vi "IntakeStateController.vi"(1 "Selected State (In)":string) -> (0 "Selected State (Out)":string)   [LabVIEW 2019]
doc: "This VI makes all decisions related to the ball intake including both intake deployment and intake speed."
uses:
  dsinstructions.vi
  outputs.vi
panel:
  in  "Intake_Speed":dbl=1.0
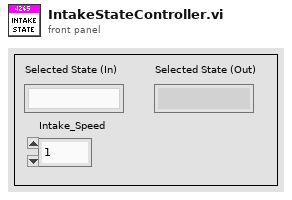
[diagram p1: front panel]
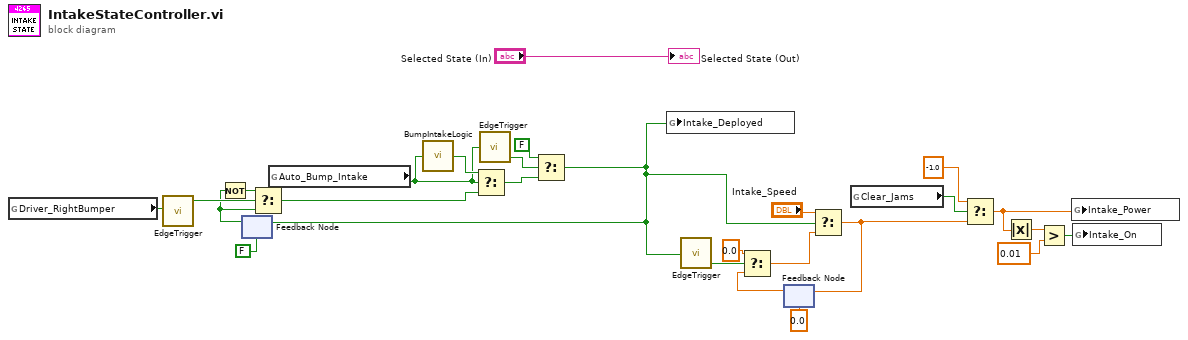
[diagram p0: block diagram]
diagram:
  n1 = global read "dsinstructions.vi" "Driver_RightBumper"() -> (w10:bool)
  n2 = call "EdgeTrigger.vi"("Input Signal"=w10) -> ("Rising Edge Trigger"=w26:bool)  [unwired: 2 out]
  n3 = feedback #1(FALSE ("Intake_On")) -> (w24:bool)
  n4 = Not(x=w24) -> (.not. x?=w23:bool)
  n5 = Select(t=w23, s=w26, f=w24) -> (s? t:f=w9:bool)
  n6 = global read "dsinstructions.vi" "Auto_Bump_Intake"() -> (w6:bool)
  n7 = call "BumpIntakeLogic.vi"("Initiate"=w6) -> ("Auto_Bump_Intake"=w8:bool)
  n8 = Select(t=w8, s=w6, f=w9) -> (s? t:f=w5:bool)
  n9 = call "EdgeTrigger.vi"("Input Signal"=w6) -> ("Falling Edge Trigger"=w7:bool)  [unwired: 2 out]
  n10 = Select(t=FALSE, s=w7, f=w5) -> (s? t:f=w2:bool)
  n11 = feedback-in #1(w2) -> ()
  n12 = global write "outputs.vi" "Intake_Deployed"(w2) -> ()
  n13 = call "EdgeTrigger.vi"("Input Signal"=w2) -> ("Falling Edge Trigger"=w20:bool)  [unwired: 2 out]
  n14 = feedback #2(0.0 ("f")) -> (w18:dbl)
  n15 = Select(t=0.0, s=w20, f=w18) -> (s? t:f=w3:dbl)
  n16 = Select(t="Intake_Speed", s=w2, f=w3) -> (s? t:f=w1:dbl)
  n17 = feedback-in #2(w1) -> ()
  n18 = global read "dsinstructions.vi" "Clear_Jams"() -> (w16:bool)
  n19 = Select(t=-1.0, s=w16, f=w1) -> (s? t:f=w14:dbl)
  n20 = Absolute Value(x=w14) -> (abs(x)=w13:dbl)
  n21 = Greater?(x=w13, y=0.01) -> (0:w11:bool)
  n22 = global write "outputs.vi" "Intake_Power"(w14) -> ()
  n23 = global write "outputs.vi" "Intake_On"(w11) -> ()
  "Selected State (Out)" <- "Selected State (In)"
